vi "update.cache.vi"(8 "error in":errorcluster, 11 "Run in":refnum<class "Run.lvclass">) -> (0 "error out":errorcluster, 3 "Run out":refnum<class "Run.lvclass">)   [LabVIEW 2020, in "Run.lvclass"]
uses:
  Run.lvclass
  Run.lvclass/Run.ctl
  2e04f76b-109b-4d14-b7ec-d7e40504a2c1.vi
  Nominal Client/Nominal Client.lvclass
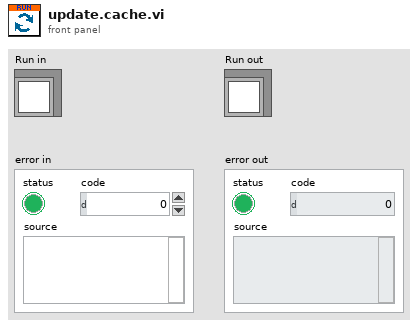
[diagram p1: front panel]
types:
  T1 = cluster{"rid":string, "runNumber":i32, "title":string, "description":string, "startTime":cluster{"secondsSinceEpoch":i32, "offsetNanoseconds":i32}, "properties":map{string, cluster{"url":string, "title":string}[]}, "labels":string[], "links":cluster{"url":string, "title":string}[], "createdAt":string, "updatedAt":string, "attachments":string[], "assets":string[], "runPrefix":string, "authorRid":string, "endTime":cluster{"secondsSinceEpoch":i32, "offsetNanoseconds":i32}, "asset":string}
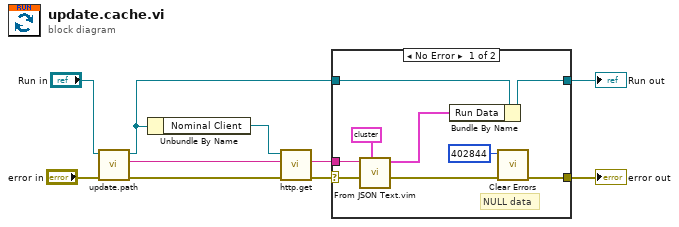
[diagram p0: block diagram]
diagram:
  n1 = call "update.path.vi"("error in"="error in", "Run"="Run in") -> ("error out"=w4:errorcluster, "path"=w8:string, "Run Out"=w10:refnum<class "Run.lvclass">)  [unwired: 7 in]
  n2 = Unbundle By Name(w10) -> ("Nominal Client"=w9:refnum<class "Nominal Client.lvclass">)
  n3 = call "http.get.vi"("error in"=w4, "Path"=w8, "Nominal Client in"=w9) -> ("error out"=w2:errorcluster, "Response"=w7:string)  [unwired: 5 in, 2 out]
  n4 = case shown="No Error" w2 {
    selector: w2 -> [w12 w21]
    tunnel: w10 -> [w15 w20]
    tunnel: w7 -> [w14 _]
    tunnel: [w13 w20] -> w6
    tunnel: [w11 w21] -> w1
    frame No Error {
      # "NULL data"
      n5 = call "From JSON Text.vim"("Data Type and Default Value"=T1 {"rid"="", "runNumber"=0, "title"="", "description"="", "startTime"={"secondsSinceEpoch"=0, "offsetNanoseconds"=0}, "properties"={}, "labels"=[], "links"=[], "createdAt"="", "updatedAt"="", "attachments"=[], "assets"=[], "runPrefix"="", "authorRid"="", "endTime"={"secondsSinceEpoch"=0, "offsetNanoseconds"=0}, "asset"=""} ("Response"), "error in (no error)"=w12, "JSON"=w14) -> ("error out"=w18:errorcluster, "Data out"=w16:T1)  [unwired: 7 in]
      n6 = Bundle By Name(cluster=w15, "Run Data"=w16) -> (w13:refnum<class "Run.lvclass">)
      n7 = call <vilib>:"Clear Errors.vi"("error in (no error)"=w18, "specific error code to clear (0: all)"=402844) -> ("error out"=w11:errorcluster)  [unwired: 4 in, 1 out]
    }
    frame Error {
    }
  }
  "Run out" <- w6
  "error out" <- w1
